vi "Set_motors_led.vi"(6 "error in (no error)":errorcluster, 8 "Color m6":T1(ring), 9 "Color m5":T1(ring), 10 "Color m3":T1(ring), 11 "Color m2":T1(ring)) -> (0 "error out":errorcluster)   [LabVIEW 2017]
uses:
  IP Address.vi
  <vilib>/httpClient/LabVIEWHTTPClient.lvlib
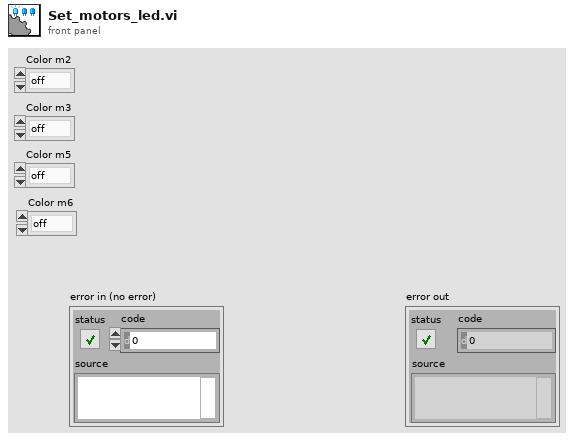
[diagram p1: front panel]
types:
  T1 = enum16{"off", "red", "green", "yellow", "blue", "pink", "cyan", "white"}
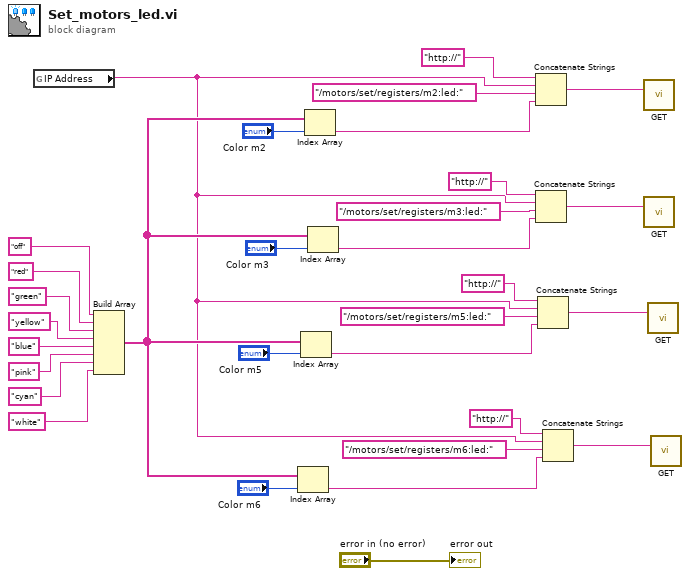
[diagram p0: block diagram]
diagram:
  n1 = global read "IP Address.vi" "IP Address"() -> (w1:string)
  n2 = Build Array("off", "red", "green", "yellow", "blue", "pink", "cyan", "white") -> (w9:string[])
  n3 = Index Array(array=w9, index="Color m6") -> (element=w6:string)
  n4 = Index Array(array=w9, index="Color m5") -> (element=w8:string)
  n5 = Index Array(array=w9, index="Color m2") -> (element=w13:string)
  n6 = Index Array(array=w9, index="Color m3") -> (element=w7:string)
  n7 = Concatenate Strings("http://" ("string"), w1, "/motors/set/registers/m2:led:" ("url"), w13) -> (w30:string)
  n8 = Concatenate Strings("http://" ("string"), w1, "/motors/set/registers/m3:led:" ("url"), w7) -> (w29:string)
  n9 = Concatenate Strings("http://" ("string"), w1, "/motors/set/registers/m5:led:" ("url"), w8) -> (w26:string)
  n10 = Concatenate Strings("http://" ("string"), w1, "/motors/set/registers/m6:led:" ("url"), w6) -> (w25:string)
  n11 = call <vilib>:"GET.vi"("url"=w30) -> ()  [unwired: 11 in, 4 out]
  n12 = call <vilib>:"GET.vi"("url"=w29) -> ()  [unwired: 11 in, 4 out]
  n13 = call <vilib>:"GET.vi"("url"=w26) -> ()  [unwired: 11 in, 4 out]
  n14 = call <vilib>:"GET.vi"("url"=w25) -> ()  [unwired: 11 in, 4 out]
  "error out" <- "error in (no error)"
